vi "Convert Rx Receive Data to String.vi"(0 "Rx_Data":u32[](array[numeric]), 1 "Port Number":u8, 5 "error in":errorcluster) -> (4 "String":string, 6 "error out":errorcluster)   [LabVIEW 2012, in "UART_Host_Driver.lvlib" / "UART Driver.lvclass"]
uses:
  UART Driver.lvclass
  FPGA/UART/UART_Response.ctl
  FPGA/UART/Parity.ctl
  FPGA/UART/StopBits.ctl
  FPGA/UART/UART_Firmware.lvlib
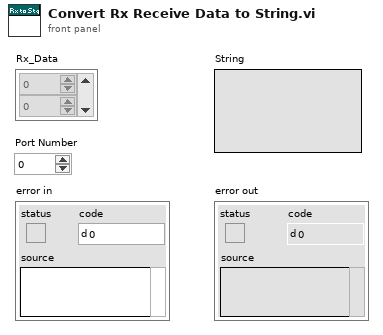
[diagram p1: front panel]
types:
  T1 = typedef "UART_Firmware.lvlib/UART_Response.ctl" = enum8{"None", "Rx", "BaudHighAck", "BaudLowAck", "CharSizeAck", "ParityAck", "StopBitsAck", "SpacingHighAck", "SpacingLowAck", "ParityError", "FrameError"}
  T2 = typedef "UART_Firmware.lvlib/Parity.ctl" = enum8{"None", "Even", "Odd"}
  T3 = typedef "UART_Firmware.lvlib/StopBits.ctl" = enum8{"1.0", "1.5", "2.0"}
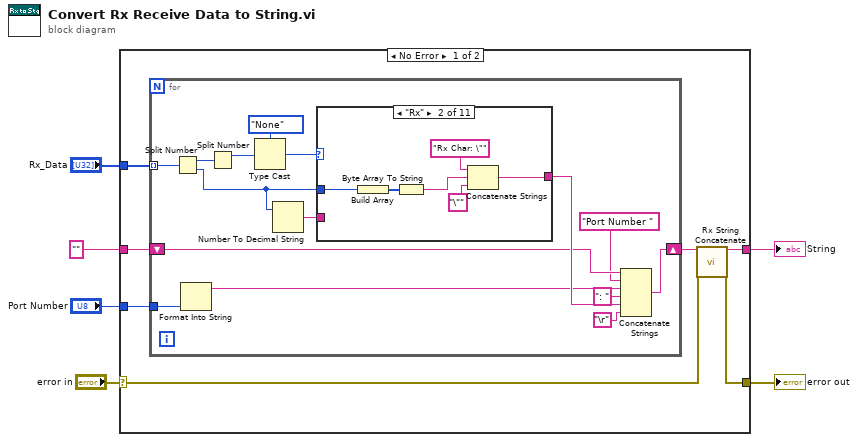
[diagram p0: block diagram]
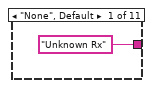
[diagram p2: hidden frame]
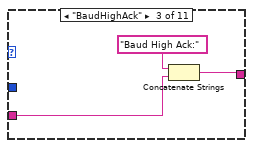
[diagram p3: hidden frame]
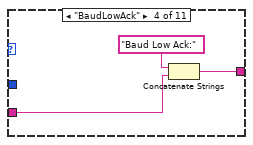
[diagram p4: hidden frame]
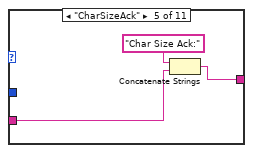
[diagram p5: hidden frame]
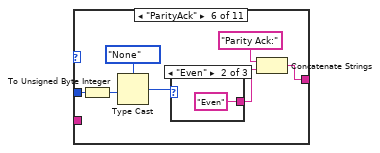
[diagram p6: hidden frame]
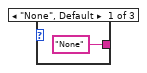
[diagram p7: hidden frame]
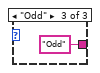
[diagram p8: hidden frame]
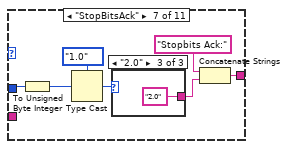
[diagram p9: hidden frame]
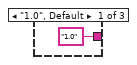
[diagram p10: hidden frame]
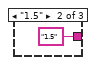
[diagram p11: hidden frame]
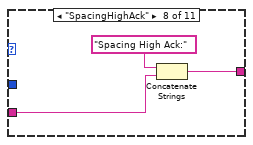
[diagram p12: hidden frame]
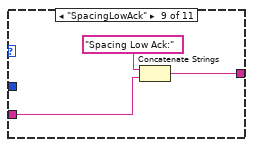
[diagram p13: hidden frame]
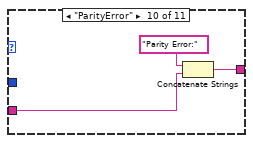
[diagram p14: hidden frame]
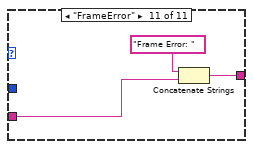
[diagram p15: hidden frame]
diagram:
  n1 = case shown="No Error" "error in" {
    selector: "error in" -> [w8 w78]
    tunnel: "" -> [w13 w77]
    tunnel: [w9 w77] -> w5
    tunnel: "Rx_Data" -> [w12 _]
    tunnel: [w7 w78] -> w2
    tunnel: "Port Number" -> [w11 _]
    frame No Error {
      n2 = for {
        tunnel: w12 -> [w28] mode=indexing
        shift-right: [w24] -> w10
        shift-left: w13 -> [w17]
        tunnel: w11 -> [w18]
        n3 = Split Number(x=w28) -> (hi(x)=w27:u16, lo(x)=w21:u16)
        n4 = Format Into String(w18) -> (resulting string=w16:string)  [unwired: 3 in, 1 out]
        n5 = Split Number(x=w27) -> (hi(x)=w26:u8)  [unwired: 1 out]
        n6 = Type Cast(type=UART_Response."None" ("UART Reply"), x=w26) -> (*(type *) &x=w25:T1)
        n7 = Number To Decimal String(number=w21) -> (decimal integer string=w20:string)  [unwired: 1 in]
        n8 = case shown="\"Rx\"" w25 {
          tunnel: w21 -> [_ w35 _ _ _ w47 w56 _ _ _ _]
          tunnel: ["Unknown Rx" w30 w36 w39 w42 w50 w58 w65 w68 w72 w75] -> w23
          tunnel: w20 -> [_ _ w37 w40 w43 _ _ w66 w69 w71 w74]
          frame "None", Default {
          }
          frame "Rx" {
            n9 = Build Array(w35) -> (w34:u16[])
            n10 = Byte Array To String(unsigned byte array=w34) -> (string=w32:string)
            n11 = Concatenate Strings("Rx Char: \"" ("string"), w32, "\"" ("string")) -> (w30:string)
          }
          frame "BaudHighAck" {
            n12 = Concatenate Strings("Baud High Ack:" ("string"), w37) -> (w36:string)
          }
          frame "BaudLowAck" {
            n13 = Concatenate Strings("Baud Low Ack:" ("string"), w40) -> (w39:string)
          }
          frame "CharSizeAck" {
            n14 = Concatenate Strings("Char Size Ack:" ("string"), w43) -> (w42:string)
          }
          frame "ParityAck" {
            n15 = To Unsigned Byte Integer(number=w47) -> (unsigned 8bit integer=w46:u8)
            n16 = Type Cast(type=Parity."None" ("Parity"), x=w46) -> (*(type *) &x=w49:T2)
            n17 = case shown="\"Even\"" w49 {
              tunnel: ["None" ("string") "Even" ("string") "Odd" ("string")] -> w48
              frame "None", Default {
              }
              frame "Even" {
              }
              frame "Odd" {
              }
            }
            n18 = Concatenate Strings("Parity Ack:" ("string"), w48) -> (w50:string)
          }
          frame "StopBitsAck" {
            n19 = To Unsigned Byte Integer(number=w56) -> (unsigned 8bit integer=w57:u8)
            n20 = Type Cast(type=StopBits."1.0" ("Stop Bits"), x=w57) -> (*(type *) &x=w60:T3)
            n21 = case shown="\"2.0\"" w60 {
              tunnel: ["1.0" ("string") "1.5" ("string") "2.0" ("string")] -> w59
              frame "1.0", Default {
              }
              frame "1.5" {
              }
              frame "2.0" {
              }
            }
            n22 = Concatenate Strings("Stopbits Ack:" ("string"), w59) -> (w58:string)
          }
          frame "SpacingHighAck" {
            n23 = Concatenate Strings("Spacing High Ack:" ("string"), w66) -> (w65:string)
          }
          frame "SpacingLowAck" {
            n24 = Concatenate Strings("Spacing Low Ack:" ("string"), w69) -> (w68:string)
          }
          frame "ParityError" {
            n25 = Concatenate Strings("Parity Error:" ("string"), w71) -> (w72:string)
          }
          frame "FrameError" {
            n26 = Concatenate Strings("Frame Error: " ("string"), w74) -> (w75:string)
          }
        }
        n27 = Concatenate Strings(w17, "Port Number " ("string"), w16, ": ", w23, "\r") -> (w24:string)
      }
      n28 = call "Rx String Concatenate.vi"("Input Rx Message"=w10, "error in"=w8) -> ("Output Rx Message"=w9:string, "error out"=w7:errorcluster)  [unwired: 12 in]
    }
    frame Error {
    }
  }
  "String" <- w5
  "error out" <- w2
